vi "SC TCP Run Sequence Command.vi"(8 "error in (no error)":errorcluster, 10 "timeout (ms)":i32, 11 "TCP Network Connection in":refnum<k5>) -> (0 "error out":errorcluster, 3 "Return":T1)   [LabVIEW 2018]
uses:
  SC TCP SequenceRun.ctl
  SC TCP StepResult.ctl
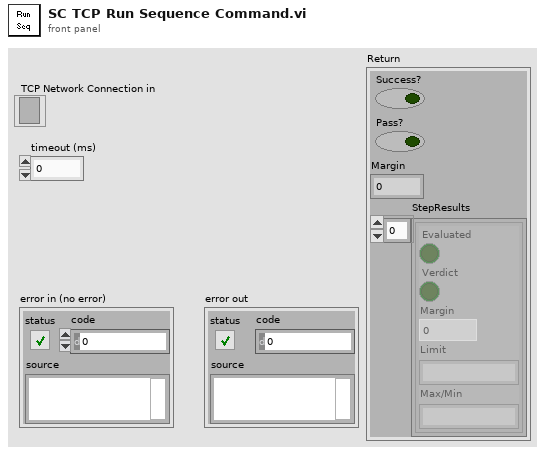
[diagram p1: front panel]
types:
  T1 = typedef "SC TCP SequenceRun.ctl" = cluster{"Success?":bool, "Pass?":bool, "Margin":dbl, "StepResults":T2[]}
  T2 = typedef "SC TCP StepResult.ctl" = cluster{"Evaluated":bool, "Verdict":bool, "Margin":dbl, "Limit":string, "Max/Min":string}
  T3 = cluster{"cmdCompleted":bool, "returnType":string, "errorType":string, "errorDescription":string, "originalCommand":string, "resolvedCommand":string}
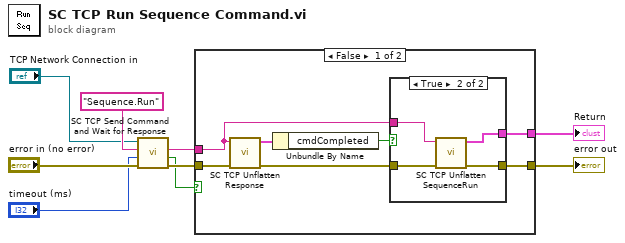
[diagram p0: block diagram]
diagram:
  n1 = call "SC TCP Send Command and Wait for Response.vi"("error in (no error)"="error in (no error)", "timeout (10000 ms)"="timeout (ms)", "Command"="Sequence.Run", "TCP Network Connection in"="TCP Network Connection in") -> ("error out"=w8:errorcluster, "Timed Out"=w3:bool, "Response"=w2:string)  [unwired: 4 in, 1 out]
  n2 = case shown="False" w3 {
    tunnel: [w16 w22] -> w9
    tunnel: [w15 _] -> w1
    tunnel: w2 -> [w13 _]
    tunnel: w8 -> [w11 w22]
    frame False {
      n3 = call "SC TCP Unflatten Response.vi"("error in"=w11, "Response JSON"=w13) -> ("error out"=w12:errorcluster, "Response Details"=w10:T3)  [unwired: 8 in]
      n4 = Unbundle By Name(w10) -> ("cmdCompleted"=w14:bool)
      n5 = case shown="True" w14 {
        tunnel: w12 -> [w17 w21]
        tunnel: w13 -> [_ w20]
        tunnel: [_ w19] -> w15
        tunnel: [w17 w18] -> w16
        frame False {
        }
        frame True {
          n6 = call "SC TCP Unflatten SequenceRun.vi"("error in"=w21, "Response JSON"=w20) -> ("error out"=w18:errorcluster, "Return"=w19:T1)  [unwired: 8 in]
        }
      }
    }
    frame True {
    }
  }
  "error out" <- w9
  "Return" <- w1
